vi "ToViewQueue.vi"(7 "Enum":T1, 8 "error in (no error)":errorcluster) -> (0 "error out":errorcluster, 3 "queue out":refnum<queue>)   [LabVIEW 2021]
uses:
  QueueEnum.ctl
  ToViewQueueData.ctl
  ViewUpdateEnum.ctl
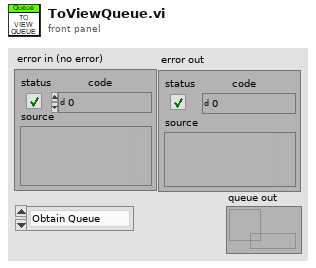
[diagram p1: front panel]
types:
  T1 = typedef "QueueEnum.ctl" = enum16{"Obtain Queue", "Get Queue Ref", "Flush Queue", "Release Queue"}
  T2 = typedef "ToViewQueueData.ctl" = cluster{"DataToUpdate":T3, "ConnectionStatus":bool, "GraphData":dbl[][], "Message":string}
  T3 = typedef "ViewUpdateEnum.ctl" = enum16{"Init", "OneButtonMessage", "Exit", "UpdateButtonsEnabled", "UpdateGraph", "UpdateConnectionStatus"}
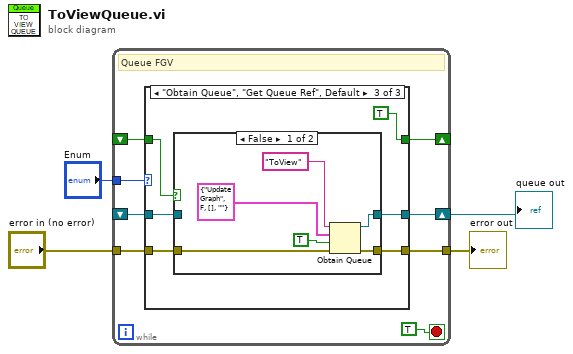
[diagram p0: block diagram]
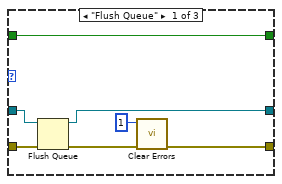
[diagram p2: hidden frame]
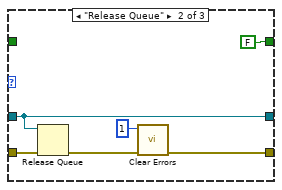
[diagram p3: hidden frame]
diagram:
  n1 = while {
    tunnel: "error in (no error)" -> [w10]
    tunnel: [w9] -> w3
    tunnel: "Enum" -> [w11]
    shift-right: [w8] -> w1
    shift-left: _ -> [w7]
    shift-right: [w6] -> _
    shift-left: _ -> [w5]
    stop <- TRUE stop-if-true
    # "Queue FGV"
    n2 = case shown="\"Obtain Queue\", \"Get Queue Ref\", Default" w11 {
      tunnel: w10 -> [w18 w25 w31]
      tunnel: [w14 w21 w30] -> w9
      tunnel: [w16 w23 w29] -> w8
      tunnel: w7 -> [w19 w23 w26]
      tunnel: [w15 FALSE TRUE] -> w6
      tunnel: w5 -> [w15 _ w27]
      frame "Flush Queue" {
        n3 = Flush Queue(queue=w19, error in (no error)=w18) -> (queue out=w16:refnum<queue>, error out=w17:errorcluster)  [unwired: 1 out]
        n4 = call <vilib>:"Clear Errors.vi"("error in (no error)"=w17, "specific error code to clear (0: all)"=1) -> ("error out"=w14:errorcluster)  [unwired: 4 in, 1 out]
      }
      frame "Release Queue" {
        n5 = Release Queue(queue=w23, error in (no error)=w25) -> (error out=w24:errorcluster)  [unwired: 1 in, 2 out]
        n6 = call <vilib>:"Clear Errors.vi"("error in (no error)"=w24, "specific error code to clear (0: all)"=1) -> ("error out"=w21:errorcluster)  [unwired: 4 in, 1 out]
      }
      frame "Obtain Queue", "Get Queue Ref", Default {
        n7 = case shown="False" w27 {
          tunnel: w31 -> [w36 w38]
          tunnel: [w34 w38] -> w30
          tunnel: [w33 w39] -> w29
          tunnel: w26 -> [_ w39]
          frame False {
            n8 = Obtain Queue(name (unnamed)="ToView", element data type=T2 {"DataToUpdate"=enum."UpdateGraph", "ConnectionStatus"=FALSE, "GraphData"=[], "Message"=""} ("ViewQueueData"), create if not found? (T)=TRUE, error in (no error)=w36) -> (queue out=w33:refnum<queue>, error out=w34:errorcluster)  [unwired: 1 in, 1 out]
          }
          frame True {
          }
        }
      }
    }
  }
  "error out" <- w3
  "queue out" <- w1
